vi "UART Open.vi"(5 "baud rate (9600)":u32=115200, 7 "parity (0:none)":enum16{"None", "Odd", "Even", "Mark", "Space"}(ring), 8 "error in":errorcluster, 11 "VISA resource name":refnum<visa-resource-name>="COM1") -> (0 "error out":errorcluster, 3 "VISA resource name out":refnum<visa-resource-name>="COM1")   [LabVIEW 2015]
uses:
  <vilib>/Instr/_visa.llb/VISA Configure Serial Port (Instr).vi
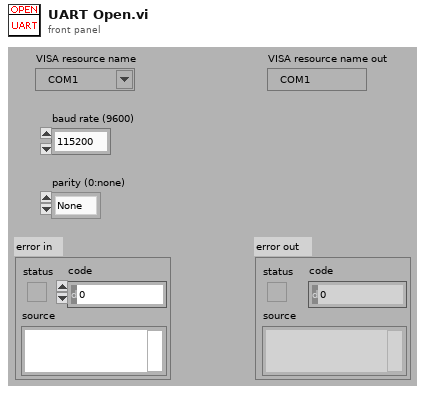
[diagram p1: front panel]
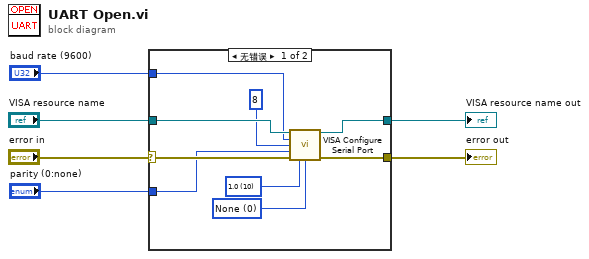
[diagram p0: block diagram]
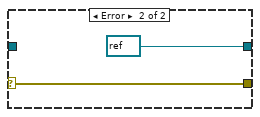
[diagram p2: hidden frame]
diagram:
  n1 = case shown="无错误" "error in" {
    selector: "error in" -> [w13 w17]
    tunnel: [w15 w17] -> w5
    tunnel: [w14 refnum<visa-resource-name> refnum ("VISA resource name out")] -> w3
    tunnel: "VISA resource name" -> [w12 _]
    tunnel: "baud rate (9600)" -> [w8 _]
    tunnel: "parity (0:none)" -> [w7 _]
    frame No Error {
      w9 = u16 0 items=["None", "XON/XOFF", "RTS/CTS", "XON/XOFF & RTS/CTS", "DTR/DSR", "XON/XOFF & DTR/DSR"] ("flow control (0:none)")
      w10 = u16 10 items=["1.0"=10, "1.5"=15, "2.0"=20] ("stop bits (10: 1 bit)")
      n2 = call-poly "VISA Configure Serial Port"("VISA resource name"=w12, "baud rate (9600)"=w8, "data bits (8)"=u16 8, "parity (0:none)"=w7, "error in (no error)"=w13, "stop bits (10: 1 bit)"=w10, "flow control (0:none)"=w9) -> ("VISA resource name out"=w14:refnum<visa-resource-name>, "error out"=w15:errorcluster)  [unwired: 7 in]
    }
    frame Error {
    }
  }
  "error out" <- w5
  "VISA resource name out" <- w3
